vi "_PC_DataChrom_Loaded_Volt.vi"(2 "dataName":string, 3 "filePath":path[](array[path])) -> (0 "Volt Value":dbl[][](array[numeric]), 1 "Plot Name":string[](array[string]))   [LabVIEW 2018]
uses:
  PublicSubVI/Class/FileManager/FM/ctl/_PC_Pub_FM fileReadFuncEnum.ctl
  PublicSubVI/Overload/Experiment Condition/_PC_Pub_ExpCondiValue_HV.vi
  PublicSubVI/Class/FileManager/TDMSAdv.lvclass
panel:
  in  "error in (no error)":errorcluster
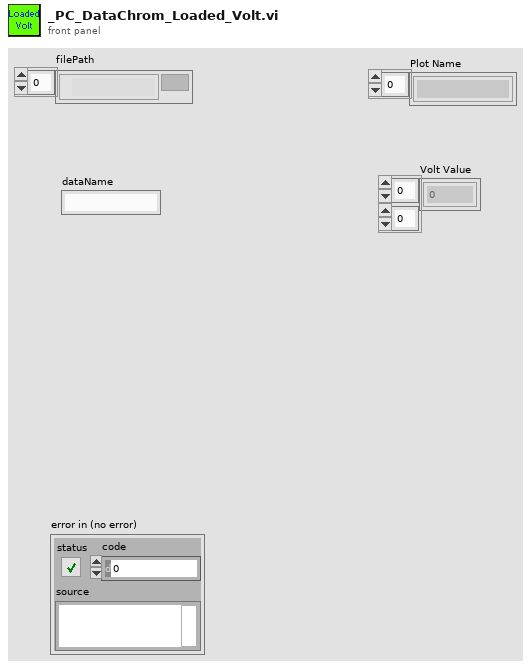
[diagram p1: front panel]
types:
  T1 = typedef "_PC_Pub_FM fileReadFuncEnum.ctl" = enum16{"getAllInfo", "getChromatogram", "getDataItems", "getTimeStamp", "getIdxData", "getIonization", "getAttrFormat"}
  T2 = enum16{"open", "open or create", "create or replace", "create", "open (read-only)"}
  T3 = typedef "_ctl_RT_D999_Format.ctl" = cluster{"Port":string, "Label":string, "Value":dbl}[]
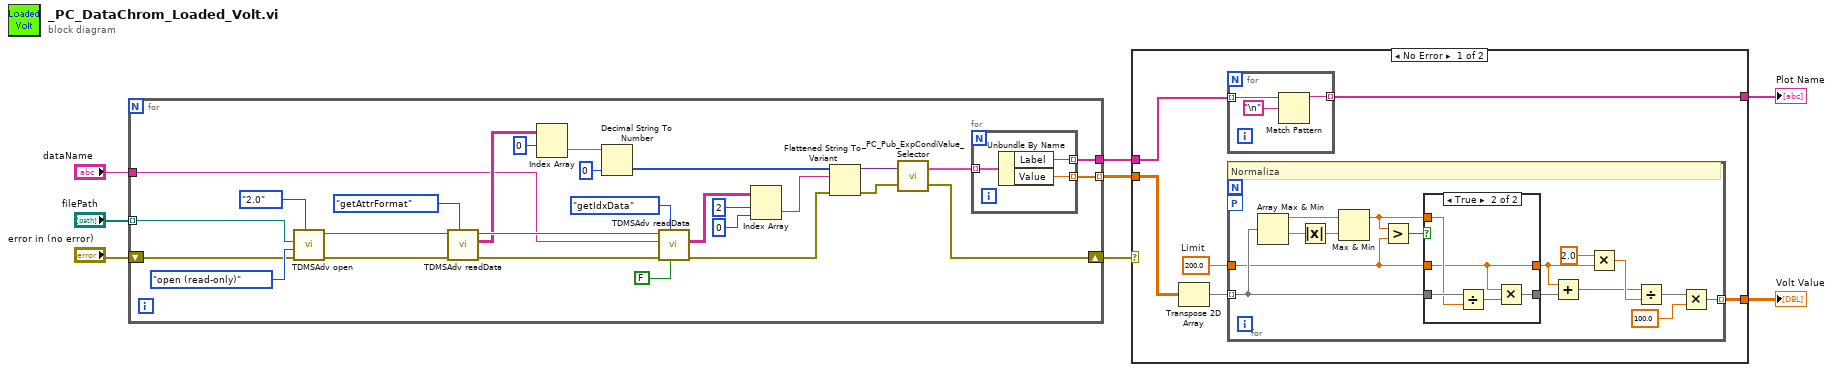
[diagram p0: block diagram]
diagram:
  n1 = for {
    tunnel: "dataName" -> [w23]
    tunnel: "filePath" -> [w22] mode=indexing
    shift-right: [w11] -> w1
    shift-left: "error in (no error)" -> [w21]
    tunnel: [w10] -> w3
    tunnel: [w9] -> w2 mode=indexing
    n2 = call "TDMSAdv open.vi"("file format version"=enum16{"1.0", "2.0", "Adv"}."2.0", "error in (no error)"=w21, "operation (0:open)"=T2."open (read-only)", "openPath"=w22) -> ("error out"=w32:errorcluster, "TDMSAdv out"=w33:refnum<class "TDMSAdv.lvclass">)  [unwired: 6 in]
    n3 = call "TDMSAdv readData.vi"("readEvent"=_PC_Pub_FM_fileReadFuncEnum."getAttrFormat", "error in (no error)"=w32, "TDMSAdv in"=w33) -> ("error out"=w29:errorcluster, "outputArr"=w24:string[][], "TDMSAdv out"=w31:refnum<class "TDMSAdv.lvclass">)  [unwired: 5 in, 1 out]
    n4 = Index Array(array=w24, index (row)=0) -> (element=w25:string[])  [unwired: 1 in]
    n5 = Decimal String To Number(string=w25, default (0L)=i16 0 ("default (0 I32)")) -> (number=w17:i16[])  [unwired: 1 in, 1 out]
    n6 = call "TDMSAdv readData.vi"("stringSplit? (T)"=FALSE, "readEvent"=_PC_Pub_FM_fileReadFuncEnum."getIdxData", "error in (no error)"=w29, "timeStamp"=w23, "TDMSAdv in"=w31) -> ("error out"=w13:errorcluster, "outputArr"=w20:string[][])  [unwired: 3 in, 2 out]
    n7 = Index Array(array=w20, index (row)=2, index (col)=0 ("disabled index (col)")) -> (element=w16:string)
    n8 = Flattened String To Variant(4:w13, 6:w16, 7:w17) -> (0:w14:errorcluster, 3:w15:variant)
    n9 = call-poly "_PC_Pub_ExpCondiValue_Selector.vi"("error in (no error)"=w14, "expCondiVariant"=w15) -> ("error out"=w11:errorcluster, "d999Value"=w12:T3)
    n10 = for {
      tunnel: w12 -> [w39] mode=indexing
      tunnel: [w38] -> w9 mode=indexing
      tunnel: [w37] -> w10 mode=indexing
      n11 = Unbundle By Name(w39) -> ("Label"=w37:string, "Value"=w38:dbl)
    }
  }
  n12 = case shown="No Error" w1 {
    tunnel: [w44 _] -> w8
    tunnel: [w43 _] -> w7
    tunnel: w3 -> [w41 _]
    tunnel: w2 -> [w40 _]
    frame No Error {
      w45 = 200.0  # Limit
      n13 = Transpose 2D Array(2D array=w40) -> (transposed array=w42:dbl[][])
      n14 = for {
        tunnel: w41 -> [w47] mode=indexing
        tunnel: [w46] -> w43 mode=indexing
        n15 = Match Pattern(string=w47, regular expression="\n") -> (before substring=w46:string)  [unwired: 1 in, 3 out]
      }
      n16 = for {
        tunnel: w42 -> [w59] mode=indexing
        tunnel: w45 -> [w56]
        tunnel: [w49] -> w44 mode=indexing
        workers-P: _ -> [_]
        # "Normaliza"
        n17 = Array Max & Min(array=w59) -> (max value=w62:dbl, min value=w63:dbl)  [unwired: 2 out]
        n18 = Absolute Value(x=w63) -> (abs(x)=w61:dbl)
        n19 = Max & Min(x=w62, y=w61) -> (max(x,y)=w58:dbl)  [unwired: 1 out]
        n20 = Greater?(x=w58, y=w56) -> (0:w60:bool)
        n21 = case shown="True" w60 {
          tunnel: w59 -> [w65 w70]
          tunnel: w58 -> [_ w69]
          tunnel: [w65 w67] -> w57
          tunnel: w56 -> [w64 w66]
          tunnel: [w64 w66] -> w55
          frame False {
          }
          frame True {
            n22 = Divide(x=w70, y=w69) -> (x/y=w68:dbl[])
            n23 = Multiply(x=w66, y=w68) -> (x*y=w67:dbl[])
          }
        }
        n24 = Add(x=w55, y=w57) -> (x+y=w52:dbl[])
        n25 = Multiply(x=2.0, y=w55) -> (x*y=w53:dbl)
        n26 = Divide(x=w52, y=w53) -> (x/y=w51:dbl[])
        n27 = Multiply(x=w51, y=100.0 ("x")) -> (x*y=w49:dbl[])
      }
    }
    frame Error {
    }
  }
  "Volt Value" <- w8
  "Plot Name" <- w7
